vi "LCR_OpenShortLoadCompensation.vi"(6 "Freq":dbl=29568.503937007874, 7 "UseCorrection":bool=TRUE, 9 "Cal Cluster":T1={"ESL_Cal"=2e-07, "ESR_Cal"=0.001, "Cp_Cal"=0.0, "Rp_Cal"=0.0, "RLoad"=1000000000.0, "RLoad_Meas"=1000000000.0} {"RLoad_Meas" format="%#_6p"; "RLoad" format="%#_6p"}, 10 "Phase Z Meas Deg":dbl=-274.14043501202957, 11 "Mag Z Meas":dbl=0.05495335386432602) -> (0 "Z DUT":cdb=0.002970463906317392-185.81585831552346i, 2 "Phase Z DUT":dbl=-89.99908406609342, 3 "Mag Z DUT":dbl=185.81585833926647)   [LabVIEW 2021]
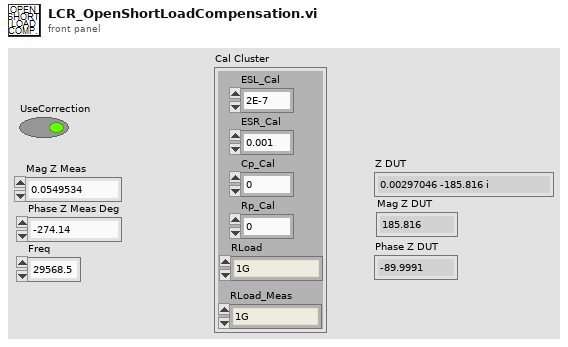
[diagram p1: front panel]
types:
  T1 = cluster{"ESL_Cal":dbl, "ESR_Cal":dbl, "Cp_Cal":dbl, "Rp_Cal":dbl, "RLoad":dbl, "RLoad_Meas":dbl}
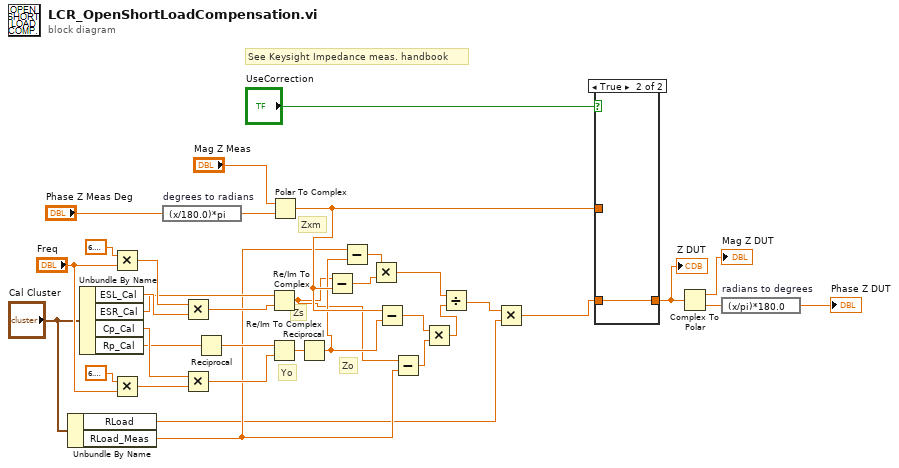
[diagram p0: block diagram]
diagram:
  # "Zo"
  # "Yo"
  # "Zxm"
  # "Zs"
  # "See Keysight Impedance meas. handbook"
  n1 = Unbundle By Name("Cal Cluster") -> ("RLoad"=w2:dbl, "RLoad_Meas"=w8:dbl)
  n2 = Unbundle By Name("Cal Cluster") -> ("ESL_Cal"=w24:dbl, "ESR_Cal"=w23:dbl, "Cp_Cal"=w20:dbl, "Rp_Cal"=w18:dbl)
  n3 = Multiply(x=6.283185307179586, y="Freq") -> (x*y=w26:dbl)
  n4 = Multiply(x=6.283185307179586, y="Freq") -> (x*y=w21:dbl)
  n5 = expression code="(x/180.0)*pi" "degrees to radians"("Phase Z Meas Deg") -> (w32:dbl)
  n6 = Multiply(x=w26, y=w24) -> (x*y=w25:dbl)
  n7 = Multiply(x=w20, y=w21) -> (x*y=w19:dbl)
  n8 = Reciprocal(x=w18) -> (1/x=w17:dbl)
  n9 = Re/Im To Complex(1:w25, 2:w23) -> (0:w9:cdb)
  n10 = Re/Im To Complex(1:w19, 2:w17) -> (0:w15:cdb)
  n11 = Polar To Complex(1:w32, 2:"Mag Z Meas") -> (0:w11:cdb)
  n12 = Reciprocal(x=w15) -> (1/x=w10:cdb)
  n13 = Subtract(x=w9, y=w11) -> (x-y=w12:cdb)
  n14 = Subtract(x=w8, y=w10) -> (x-y=w13:cdb)
  n15 = Multiply(x=w13, y=w12) -> (x*y=w4:cdb)
  n16 = Subtract(x=w11, y=w10) -> (x-y=w7:cdb)
  n17 = Subtract(x=w9, y=w8) -> (x-y=w6:cdb)
  n18 = Multiply(x=w7, y=w6) -> (x*y=w5:cdb)
  n19 = Divide(x=w4, y=w5) -> (x/y=w3:cdb)
  n20 = Multiply(x=w3, y=w2) -> (x*y=w1:cdb)
  n21 = case shown="True" "UseCorrection" {
    tunnel: w1 -> [_ w37]
    tunnel: [w36 w37] -> w30
    tunnel: w11 -> [w36 _]
    frame False {
    }
    frame True {
    }
  }
  "Z DUT" <- w30
  n22 = Complex To Polar(r * e^(i*theta)=w30) -> (r=→"Mag Z DUT":dbl, theta=w29:dbl)
  n23 = expression code="(x/pi)*180.0" "radians to degrees"(w29) -> (→"Phase Z DUT":dbl)
